vi "Init.vi"(7 "Input Data":T1, 8 "error in (no error)":errorcluster caption="错误输入（无错误）", 11 "SM Data In":T3) -> (0 "error out":errorcluster caption="错误输出", 2 "State":T2, 3 "SM Data Out":T3, 5 "State Changed":bool)   [LabVIEW 2013, in "标准状态机模板.lvlib"]
uses:
  Control/SM Data.ctl
  Control/State.ctl
  Control/Input Data.ctl
  Control/Output Data.ctl
  Control/Internal Data.ctl
  <vilib>/ptbypt/NI_PtbyPt.lvlib
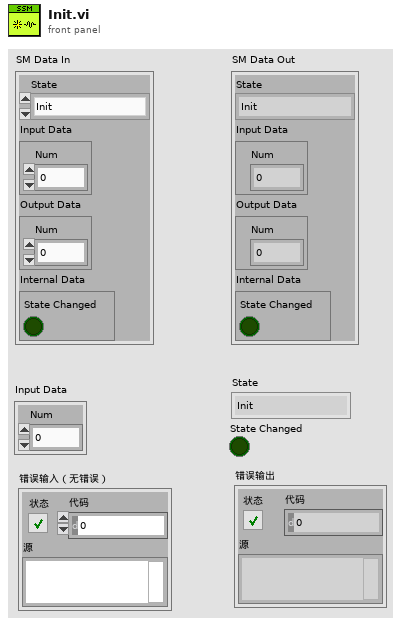
[diagram p1: front panel]
types:
  T1 = typedef "标准状态机模板.lvlib/Input Data.ctl" = cluster{"Num":dbl}
  T2 = typedef "标准状态机模板.lvlib/State.ctl" = enum16{"Init", "Idle"}
  T3 = typedef "标准状态机模板.lvlib/SM Data.ctl" = cluster{"State":T2, "Input Data":T1, "Output Data":T4, "Internal Data":T5}
  T4 = typedef "标准状态机模板.lvlib/Output Data.ctl" = cluster{"Num":dbl}
  T5 = typedef "标准状态机模板.lvlib/Internal Data.ctl" = cluster{"State Changed":bool}
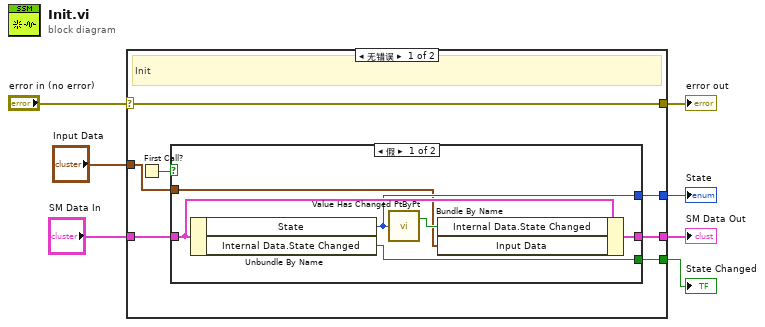
[diagram p0: block diagram]
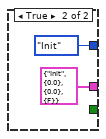
[diagram p2: hidden frame]
diagram:
  n1 = case shown="无错误" "error in (no error)" {
    selector: "error in (no error)" -> [w11 w24]
    tunnel: "SM Data In" -> [w14 w23]
    tunnel: [w13 w23] -> w5
    tunnel: [w11 w24] -> w4
    tunnel: [w10 _] -> w3
    tunnel: [w9 _] -> w2
    tunnel: "Input Data" -> [w8 _]
    frame No Error {
      # "Init"
      n2 = First Call?() -> (First Call?: T/F=w12:bool)
      n3 = case shown="假" w12 {
        tunnel: w14 -> [w19 _]
        tunnel: [w20 T3 {"State"=enum."Init", "Input Data"={"Num"=0.0}, "Output Data"={"Num"=0.0}, "Internal Data"={"State Changed"=FALSE}} ("SM Data In")] -> w13
        tunnel: [w17 State."Init" ("State")] -> w10
        tunnel: [w16 _] -> w9
        tunnel: w8 -> [w15 _]
        frame False {
          n4 = Unbundle By Name(w19) -> ("State"=w17:T2, "Internal Data.State Changed"=w16:bool)
          n5 = call <vilib>:"Value Has Changed PtByPt.vi"("input data point"=w17) -> ("has changed"=w18:bool)  [unwired: 1 in, 1 out]
          n6 = Bundle By Name(cluster=w19, "Internal Data.State Changed"=w18, "Input Data"=w15) -> (w20:T3)
        }
        frame True {
        }
      }
    }
    frame Error {
    }
  }
  "error out" <- w4
  "SM Data Out" <- w5
  "State" <- w3
  "State Changed" <- w2
